vi "Get Depth Image.vi"(8 "error in (no error)":errorcluster, 9 "Wait For Next Image?":bool=TRUE, 10 "Flip Image?":bool=TRUE, 11 "queue in":refnum<queue>) -> (0 "error out":errorcluster, 1 "Image Is New?":bool, 2 "Depth Image Pixels (U16)":u16[][](array[numeric]), 3 "Depth Image":T1(plugin-control))   [LabVIEW 2011, in "Kinect_API.lvlib"]
uses:
  Kinect_API.lvlib
  <vilib>/vision/Image Controls.llb/IMAQ Image.ctl
  <vilib>/vision/NI_Vision_Development_Module.lvlib
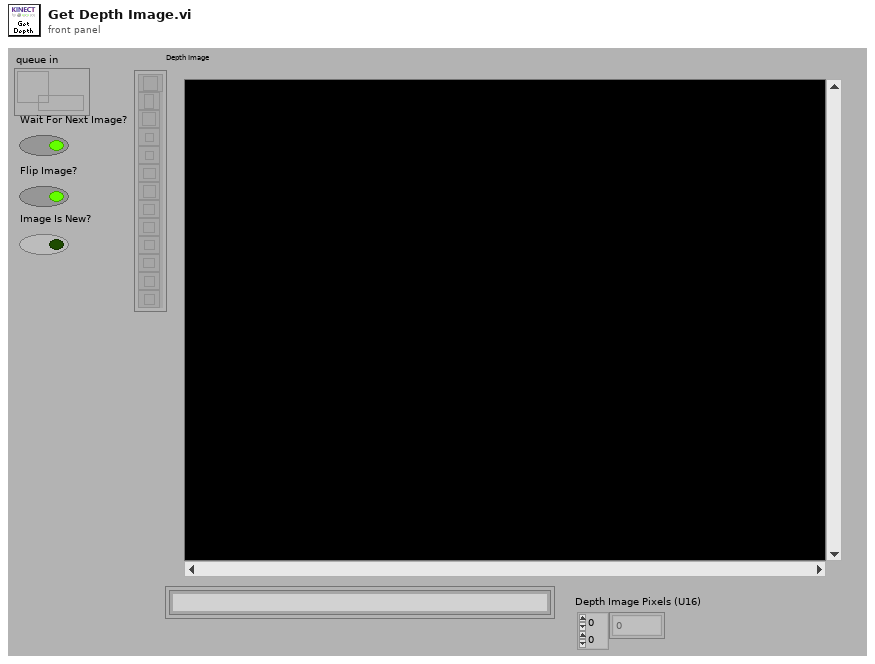
[diagram p1: front panel]
types:
  T1 = typedef "IMAQ Image.ctl" = refnum<image>
  T2 = typedef "Image Type" = u32
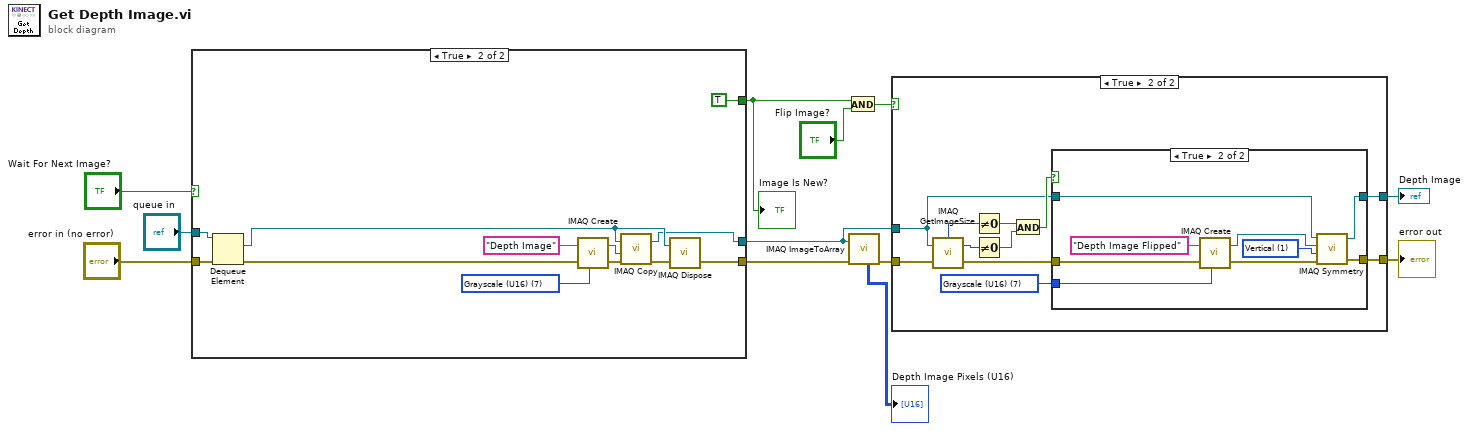
[diagram p0: block diagram]
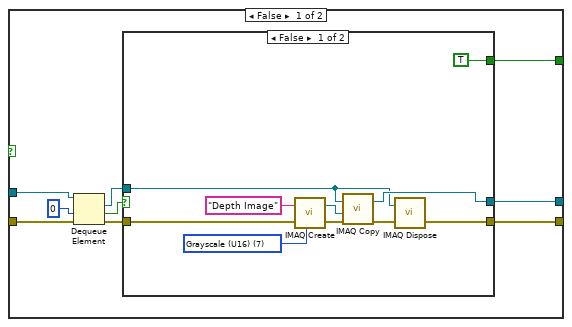
[diagram p4: hidden frame]
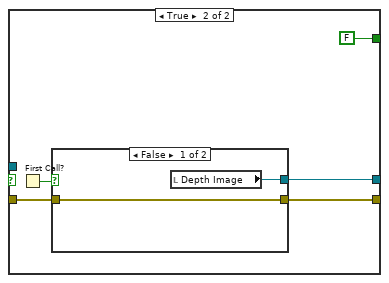
[diagram p5: hidden frame]
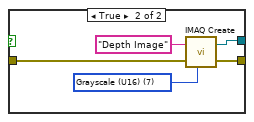
[diagram p6: hidden frame]
diagram:
  n1 = case shown="True" "Wait For Next Image?" {
    tunnel: "error in (no error)" -> [w17 w55]
    tunnel: [w19 w44] -> w5
    tunnel: [w20 w45] -> w8
    tunnel: [w21 TRUE] -> w1
    tunnel: "queue in" -> [w18 w53]
    frame False {
      n2 = Dequeue Element(queue=w18, timeout in ms (-1)=0, error in (no error)=w17) -> (element=w13:T1, timed out?=w14:bool, error out=w16:errorcluster)  [unwired: 1 out]
      n3 = case shown="False" w14 {
        tunnel: [w27 w34] -> w19
        tunnel: w16 -> [w22 w33]
        tunnel: [w24 w32] -> w20
        tunnel: [TRUE FALSE] -> w21
        tunnel: w13 -> [w23 _]
        frame False {
          w26 = T2 7 items=["Grayscale (U8)", "Grayscale (I16)", "Grayscale (SGL)", "Complex (CSG)", "RGB (U32)", "HSL (U32)", "RGB (U64)", "Grayscale (U16)"] ("Image Type")
          n4 = call "IMAQ Create"("Image Name"="Depth Image", "Image Type"=w26, "error in (no error)"=w22) -> ("New Image"=w29:T1, "error out"=w28:errorcluster)  [unwired: 2 in]
          n5 = call "IMAQ Copy"("error in (no error)"=w28, "Image Dst"=w29, "Image Src"=w23) -> ("error out"=w25:errorcluster, "Image Dst Out"=w27:T1)  [unwired: 3 in]
          n6 = call "IMAQ Dispose"("Image"=w23, "error in (no error)"=w25) -> ("error out"=w24:errorcluster)  [unwired: 4 in]
        }
        frame True {
          n7 = First Call?() -> (First Call?: T/F=w35:bool)
          n8 = case shown="False" w35 {
            tunnel: [w38 w39] -> w34
            tunnel: w33 -> [w37 w41]
            tunnel: [w37 w40] -> w32
            frame False {
              n9 = local read "Depth Image"() -> (w38:T1)
            }
            frame True {
              w42 = T2 7 items=["Grayscale (U8)", "Grayscale (I16)", "Grayscale (SGL)", "Complex (CSG)", "RGB (U32)", "HSL (U32)", "RGB (U64)", "Grayscale (U16)"] ("Image Type")
              n10 = call "IMAQ Create"("Image Name"="Depth Image", "Image Type"=w42, "error in (no error)"=w41) -> ("New Image"=w39:T1, "error out"=w40:errorcluster)  [unwired: 2 in]
            }
          }
        }
      }
    }
    frame True {
      w48 = T2 7 items=["Grayscale (U8)", "Grayscale (I16)", "Grayscale (SGL)", "Complex (CSG)", "RGB (U32)", "HSL (U32)", "RGB (U64)", "Grayscale (U16)"] ("Image Type")
      n11 = Dequeue Element(queue=w53, error in (no error)=w55) -> (element=w47:T1, error out=w51:errorcluster)  [unwired: 1 in, 2 out]
      n12 = call "IMAQ Create"("Image Name"="Depth Image", "Image Type"=w48, "error in (no error)"=w51) -> ("New Image"=w50:T1, "error out"=w49:errorcluster)  [unwired: 2 in]
      n13 = call "IMAQ Copy"("error in (no error)"=w49, "Image Dst"=w50, "Image Src"=w47) -> ("error out"=w46:errorcluster, "Image Dst Out"=w44:T1)  [unwired: 3 in]
      n14 = call "IMAQ Dispose"("Image"=w47, "error in (no error)"=w46) -> ("error out"=w45:errorcluster)  [unwired: 4 in]
    }
  }
  "Image Is New?" <- w1
  n15 = And(x=w1, y="Flip Image?") -> (x .and. y?=w2:bool)
  n16 = call "IMAQ ImageToArray"("error in (no error)"=w8, "Image"=w5) -> ("Image Pixels (U16)"=→"Depth Image Pixels (U16)":u16[][], "error out"=w4:errorcluster)  [unwired: 2 in, 3 out]
  n17 = case shown="True" w2 {
    tunnel: w5 -> [w57 w58]
    tunnel: [w57 w68] -> w7
    tunnel: w4 -> [w56 w63]
    tunnel: [w56 w67] -> w6
    frame False {
    }
    frame True {
      w66 = T2 7 items=["Grayscale (U8)", "Grayscale (I16)", "Grayscale (SGL)", "Complex (CSG)", "RGB (U32)", "HSL (U32)", "RGB (U64)", "Grayscale (U16)"] ("Image Type")
      n18 = call "IMAQ GetImageSize"("Image"=w58, "error in (no error)"=w63) -> ("Y Resolution"=w65:i32, "X Resolution"=w64:i32, "error out"=w62:errorcluster)  [unwired: 2 in]
      n19 = Not Equal To 0?(x=w64) -> (x != 0?=w61:bool)
      n20 = Not Equal To 0?(x=w65) -> (x != 0?=w60:bool)
      n21 = And(x=w61, y=w60) -> (x .and. y?=w59:bool)
      n22 = case shown="True" w59 {
        tunnel: [w70 w78] -> w68
        tunnel: [w69 w77] -> w67
        tunnel: w66 -> [_ w76]
        tunnel: w62 -> [w69 w73]
        tunnel: w58 -> [w70 w72]
        frame False {
        }
        frame True {
          w79 = u32 1 items=["Horizontal", "Vertical", "Central", "1st Diagonal", "2nd Diagonal"] ("Type of Symmetry")
          n23 = call "IMAQ Create"("Image Name"="Depth Image Flipped", "Image Type"=w76, "error in (no error)"=w73) -> ("New Image"=w75:T1, "error out"=w74:errorcluster)  [unwired: 2 in]
          n24 = call "IMAQ Symmetry"("error in (no error)"=w74, "Type of Symmetry"=w79, "Image Dst"=w75, "Image Src"=w72) -> ("error out"=w77:errorcluster, "Image Dst Out"=w78:T1)  [unwired: 1 in]
        }
      }
    }
  }
  "Depth Image" <- w7
  "error out" <- w6
